vi "Configure.vi"(8 "error in (no error)":errorcluster, 10 "Msg in":T7, 11 "FakePressureController in":refnum<class "MagAnalysis_Online.lvclass">) -> (0 "error out":errorcluster, 1 "new command":string, 2 "Msg out":T7, 3 "FakePressureController out":refnum<class "MagAnalysis_Online.lvclass">)   [LabVIEW 2020, in "MagAnalysis_Online.lvclass"]
uses:
  MagAnalysis_Online.lvclass
  DriverMsg.ctl
  CamSettingSUB_TypDEf.ctl
  CamAndObj_TypDEf.ctl
  OnOffTypeDef.ctl
  userROI.ctl
  source/Device Drivers/shared/numericVariable_TypeDef.ctl
  CamRoiTypDef.ctl
  MagAnalysis_Online.lvclass/MagAnalysis_Online.ctl
  source/Device Drivers/BaseDriver/BaseDriver.lvclass
  <resource>/objmgr/imaqdx.rc
panel:
  out "found? 2":bool
  out "found?":bool
  out "Cam 2.center":dbl
  out "Cam 1.center":dbl
  out "data":T1={"position"=0.0, "pixelsize"=0.0, "start"=0.0, "end"=0.0, "center"=0.0, "Lens"=enum."FL1-f8x08", "Forward"=enum."off", "Spec_Calib_file 2"=path "Y:/100TWdata/ESMCalib/datFwd.txt", "map"=path "Y:/100TWdata/ESMCalib/mapFwd.txt", "y size"=0, "UserROI"={"Width"={"Value"=0.0, "Min"=0.0, "Max"=0.0, "StepSize"=0.0, "Tolerance"=0.0, "ValueActual"=0.0}, "Hight"={"Value"=0.0, "Min"=0.0, "Max"=0.0, "StepSize"=0.0, "Tolerance"=0.0, "ValueActual"=0.0}, "OffsetX"={"Value"=0.0, "Min"=0.0, "Max"=0.0, "StepSize"=0.0, "Tolerance"=0.0, "ValueActual"=0.0}, "OffsetY"={"Value"=0.0, "Min"=0.0, "Max"=0.0, "StepSize"=0.0, "Tolerance"=0.0, "ValueActual"=0.0}}, "CamMaxPixel"={"X"=0, "Y"=0}, "CamROI"={"Width"=0.0, "Hight"=0.0, "OffsetX"=0.0, "OffsetY"=0.0}}
  out "Cam 0.center":dbl
  out "before substring 2":string
  out "ROI":i32[][](array[numeric])
  out "number":i32
  out "Command":string
  out "Channel":string
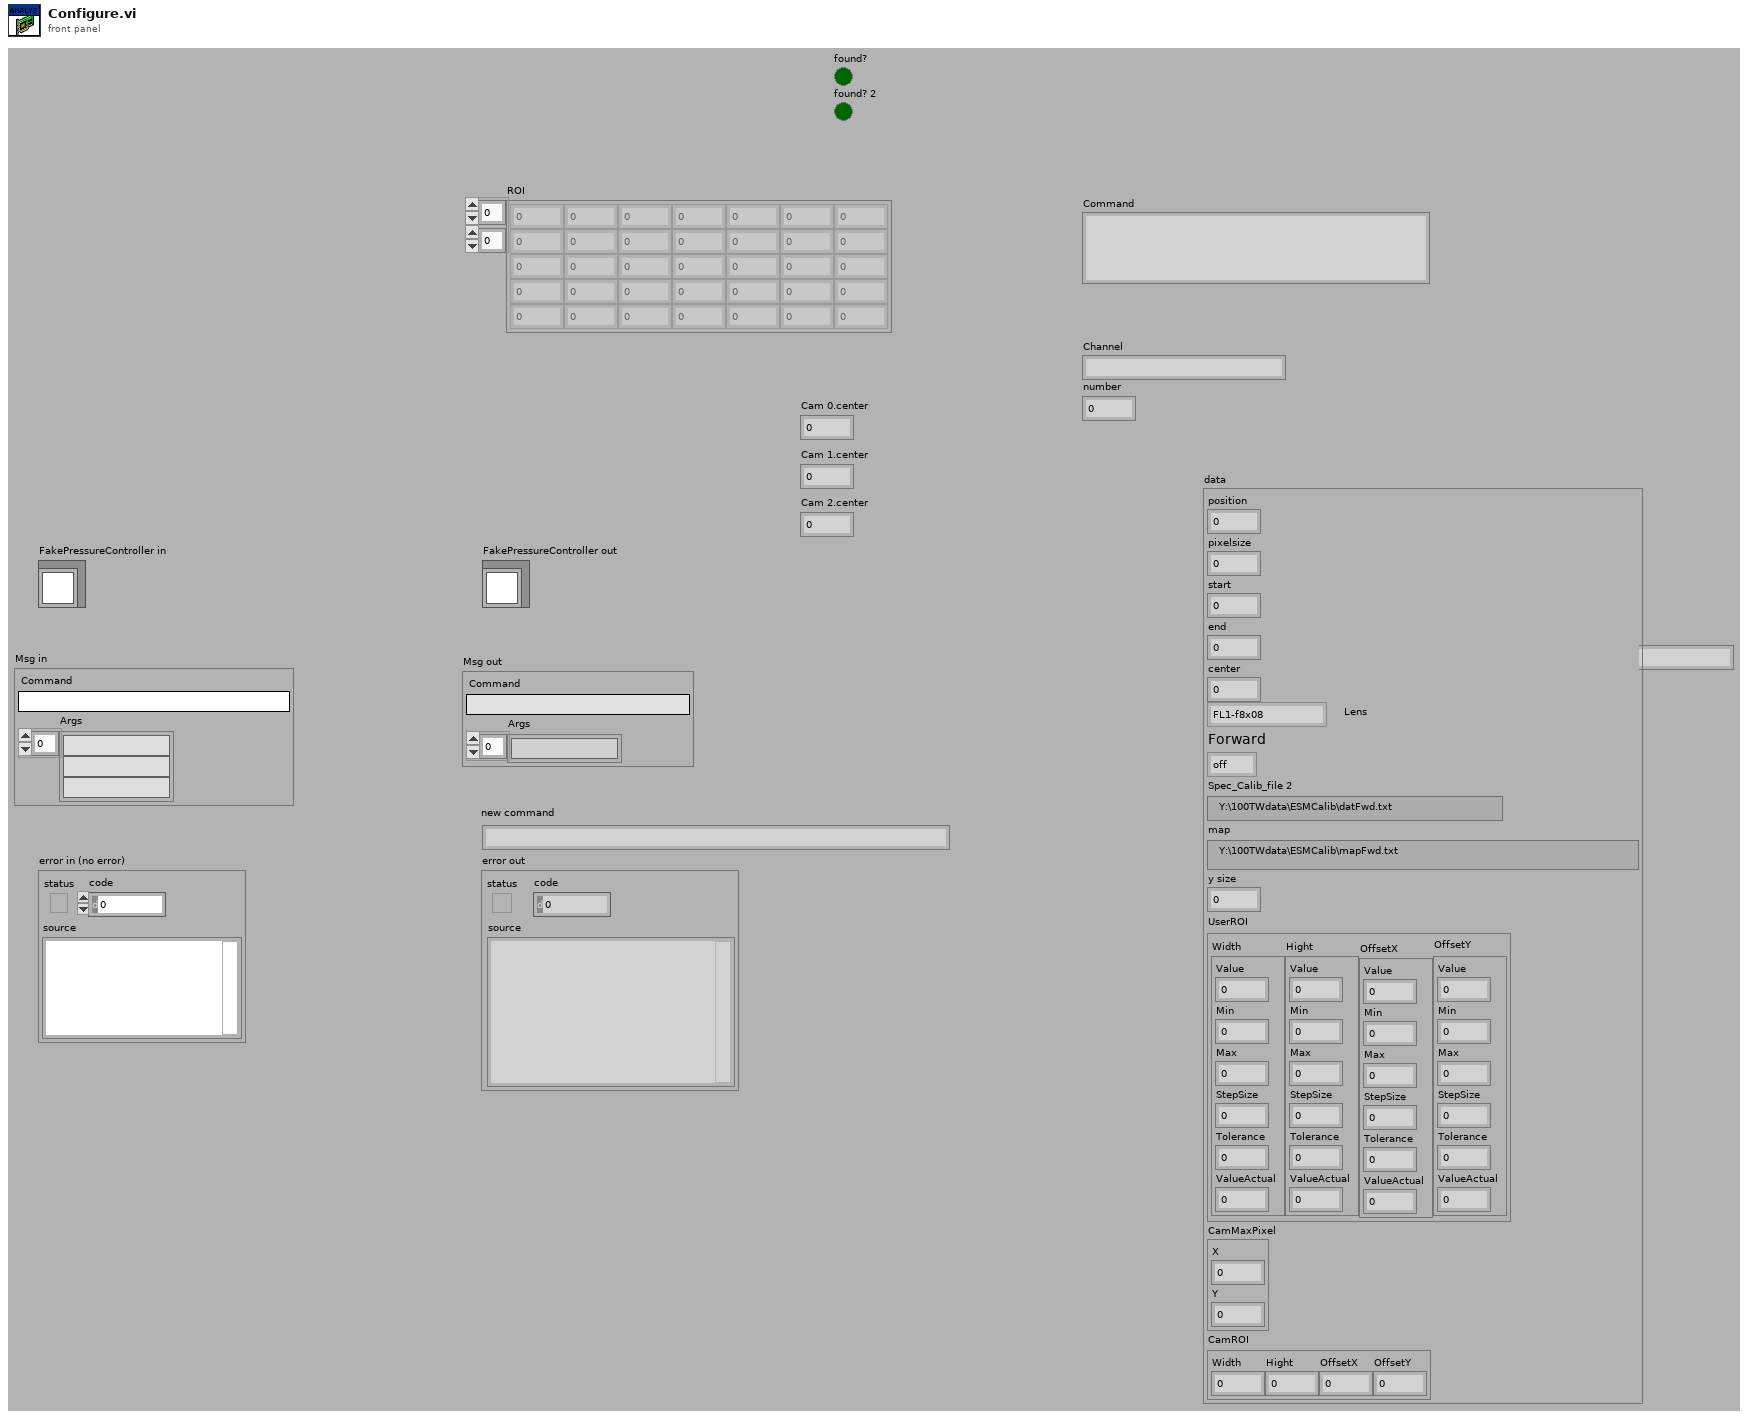
[diagram p1: front panel]
types:
  T1 = typedef "CamSettingSUB_TypDEf.ctl" = cluster{"position":dbl, "pixelsize":dbl, "start":dbl, "end":dbl, "center":dbl, "Lens":T2, "Forward":T3, "Spec_Calib_file 2":path, "map":path, "y size":i32, "UserROI":T4, "CamMaxPixel":cluster{"X":i32, "Y":i32}, "CamROI":T6}
  T2 = typedef "CamAndObj_TypDEf.ctl" = enum16{"FL1-f8x08", "FL1-f8x06", "FL1-f8", "ch300-f50", "FL2G-f8", "FL3M14-f8", "FL3M14-f8x08", "FL3M14-f8x08(2x2)"}
  T3 = typedef "OnOffTypeDef.ctl" = enum16{"off", "on"}
  T4 = typedef "userROI.ctl" = cluster{"Width":T5, "Hight":T5, "OffsetX":T5, "OffsetY":T5}
  T5 = typedef "BaseDriver.lvclass/numericVariable_TypeDef.ctl" = cluster{"Value":dbl, "Min":dbl, "Max":dbl, "StepSize":dbl, "Tolerance":dbl, "ValueActual":dbl}
  T6 = typedef "CamRoiTypDef.ctl" = cluster{"Width":dbl, "Hight":dbl, "OffsetX":dbl, "OffsetY":dbl}
  T7 = typedef "DriverMsg.ctl" = cluster{"Command":string, "Args":string[]}
  T8 = typedef "MagAnalysis_Online.lvclass/settings_TypDef.ctl" = cluster{"CamSettings":T9, "timeout":T5, "Screws":T10, "number of cam":dbl, "X size":dbl, "srewstart":T13, "Save":T3, "offset":dbl, "localsavingpath":path, "ROIString":string, "exposure":T5, "trigger":T3}
  T9 = typedef "CamSettings_Typdef.ctl" = cluster{"Cam 0":T1, "Cam 1":T1, "Cam 2":T1, "Cam 3":T1}
  T10 = typedef "SrewMaster_TYpDef.ctl" = cluster{"Cam 0":T11, "Cam 1":T11, "Cam 2":T11, "Cam 3":T11}
  T11 = typedef "srew_TypDEf.ctl" = cluster{"S 0":T12, "S 1":T12, "S 2":T12, "S 3":T12, "S 4":T12, "S 5":T12}
  T12 = typedef "ScrewSub_Typdef.ctl" = cluster{"0":i32, "1":i32, "2":i32, "3":i32}
  T13 = typedef "screwstart.ctl" = cluster{"Cam 0":dbl, "Cam 1":dbl, "Cam 2":dbl, "Cam 3":dbl}
  T14 = typedef "IMAQdx.ctl" = refnum<k21>
  T15 = cluster{"CamSettings[0]":T1, "CamSettings[1]":T1, "CamSettings[2]":T1, "CamSettings[3]":T1}
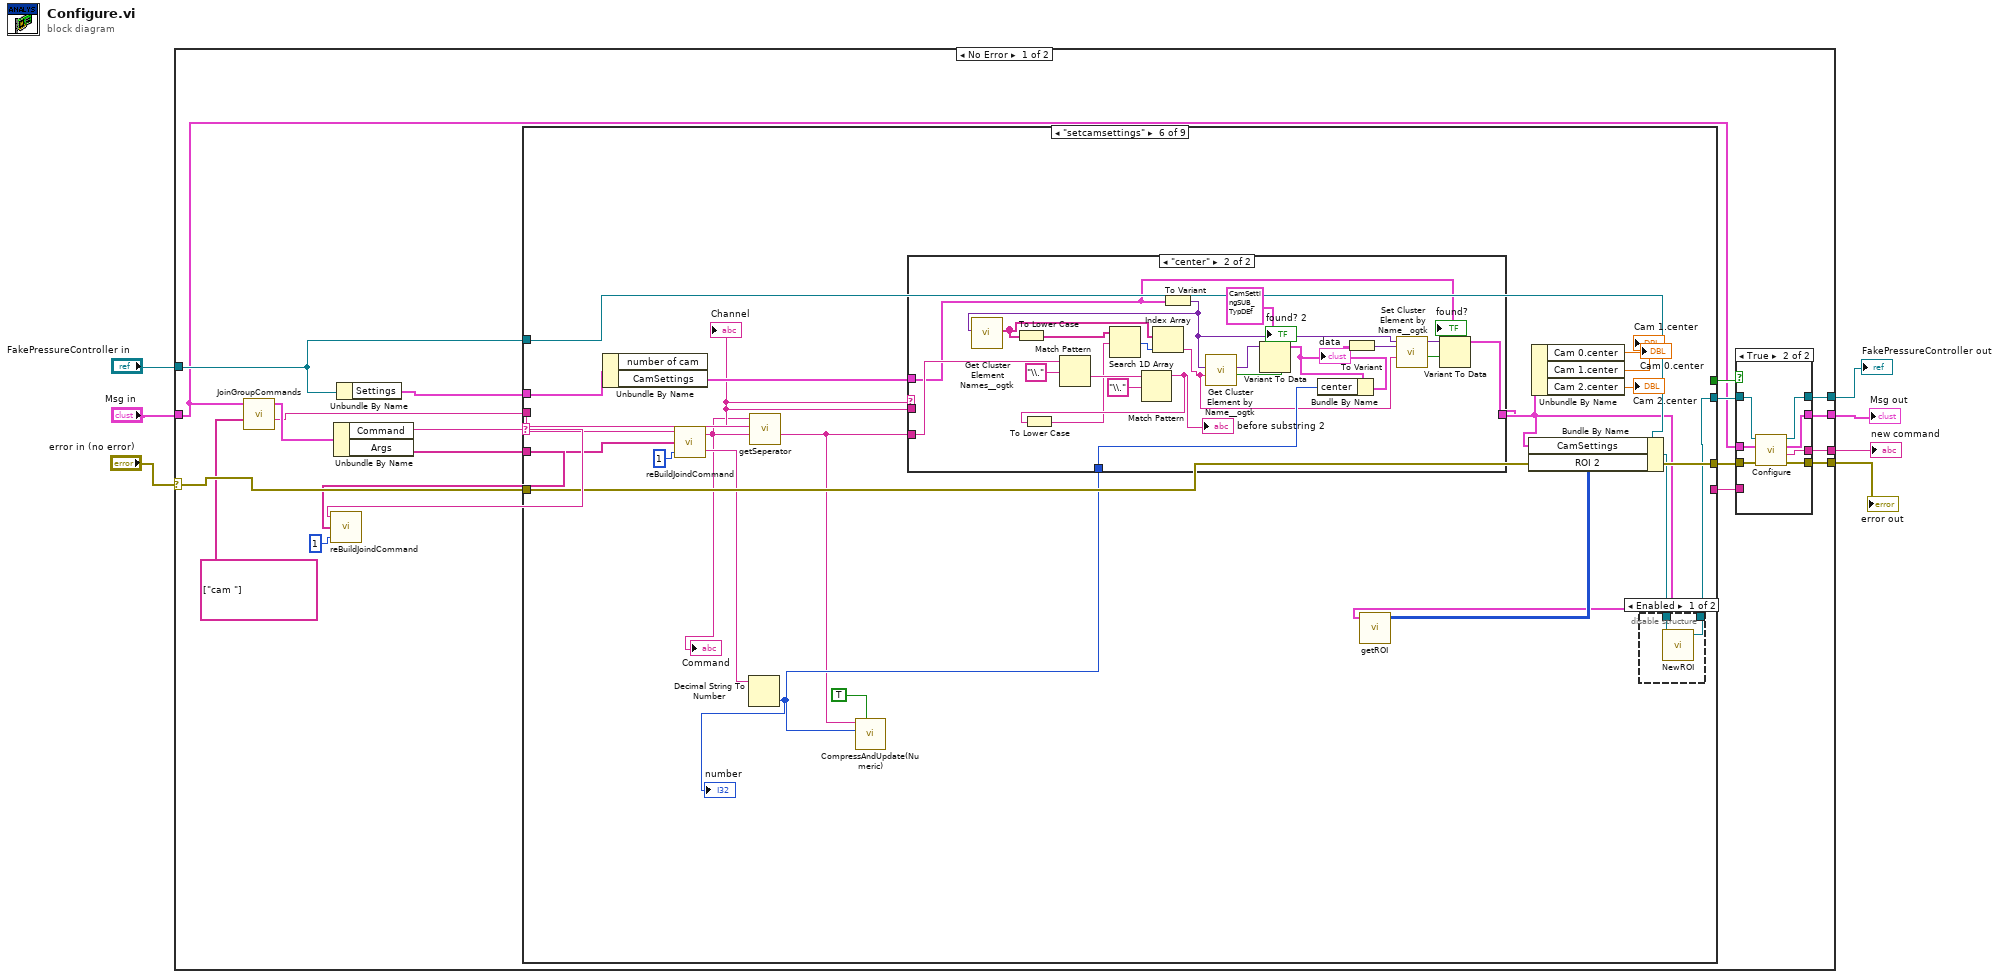
[diagram p0: block diagram]
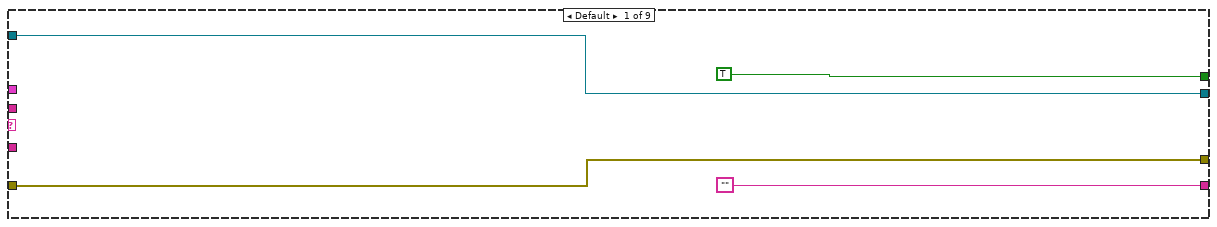
[diagram p3: hidden frame]
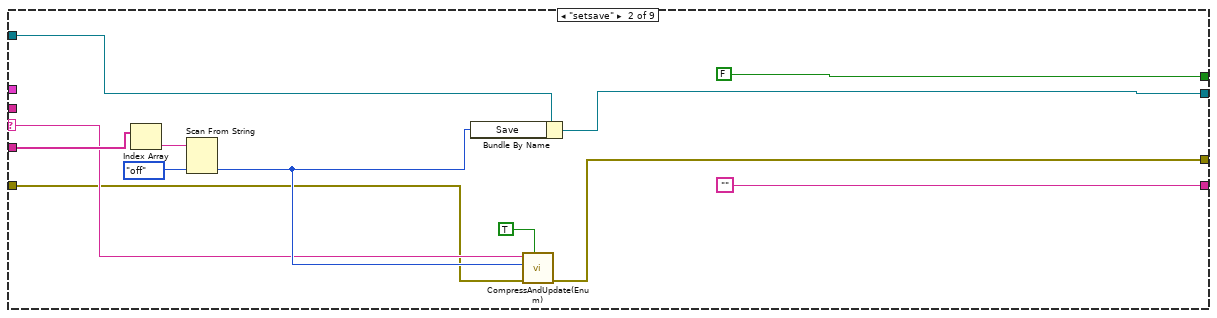
[diagram p4: hidden frame]
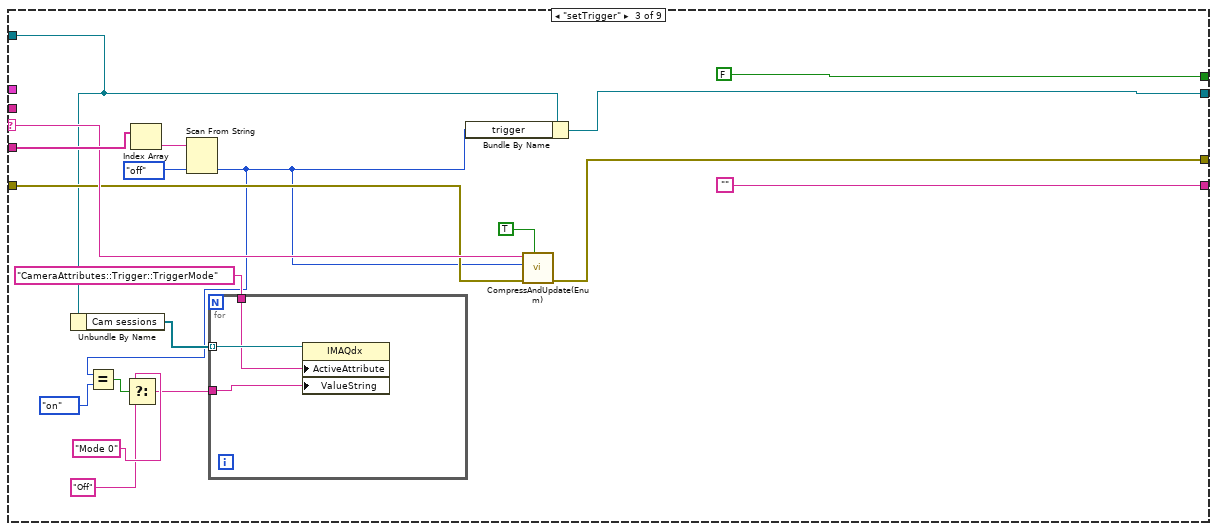
[diagram p5: hidden frame]
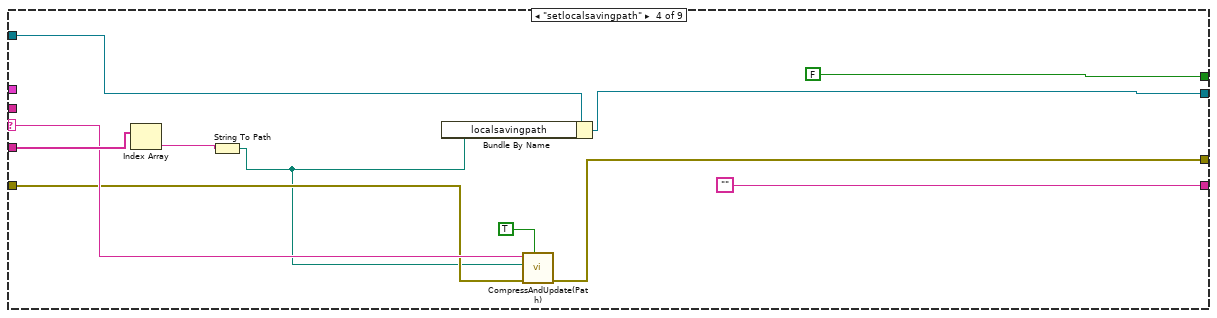
[diagram p6: hidden frame]
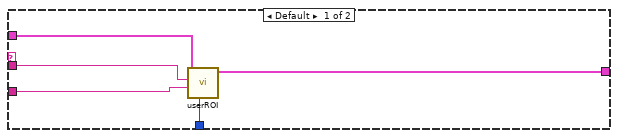
[diagram p9: hidden frame]
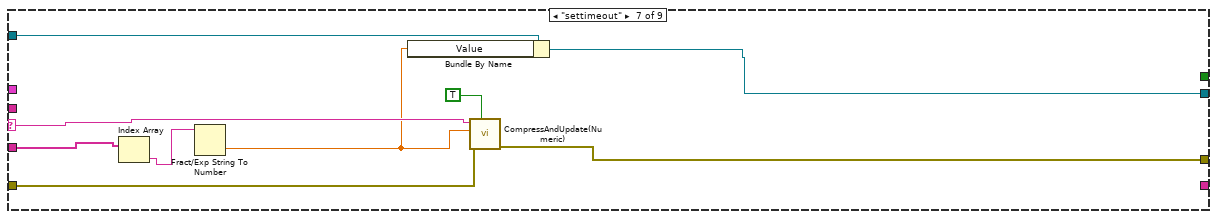
[diagram p10: hidden frame]
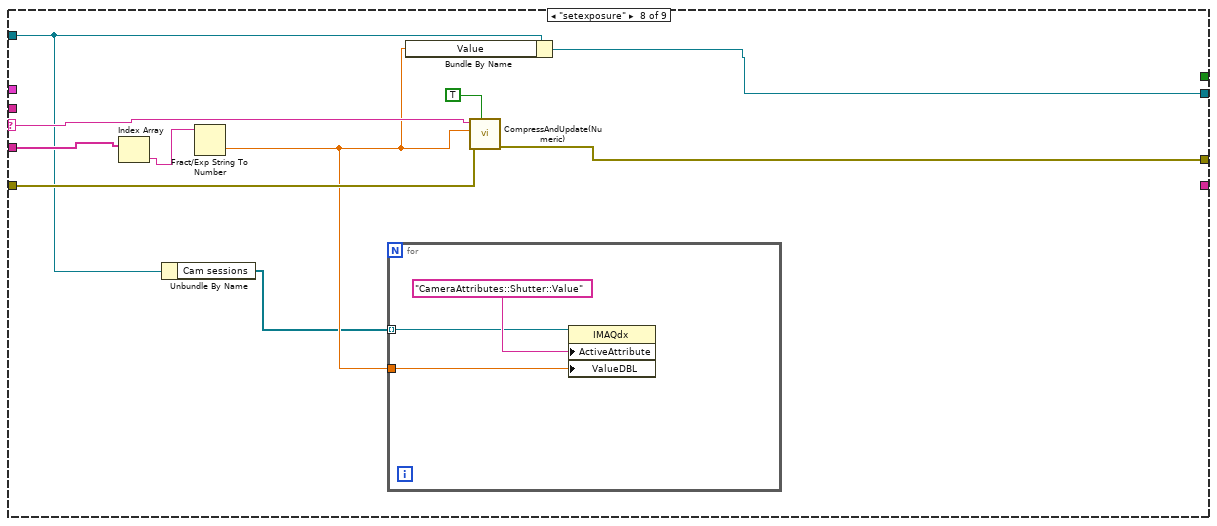
[diagram p11: hidden frame]
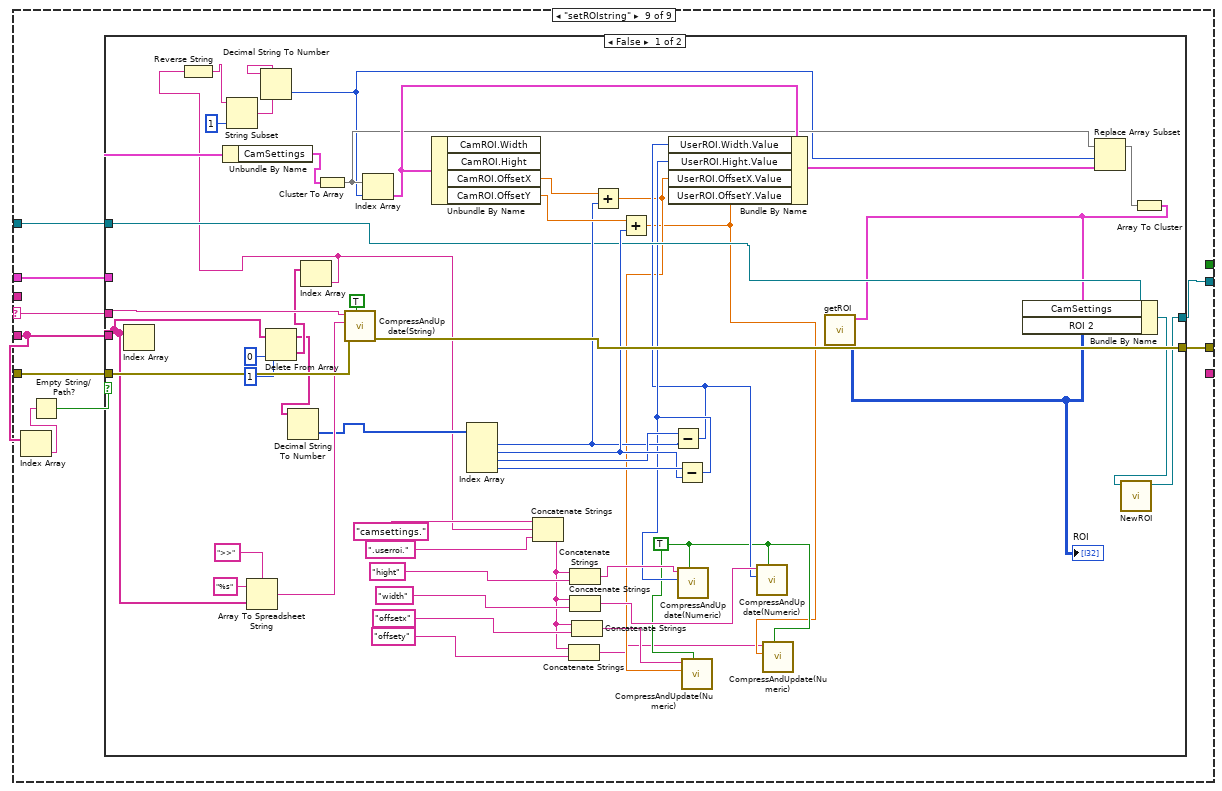
[diagram p12: hidden frame]
diagram:
  n1 = case shown="No Error" "error in (no error)" {
    selector: "error in (no error)" -> [w16 w224]
    tunnel: "FakePressureController in" -> [w17 w222]
    tunnel: [w24 w222] -> w4
    tunnel: [w22 w224] -> w1
    tunnel: "Msg in" -> [w15 w223]
    tunnel: [w20 w223] -> w3
    tunnel: [w18 _] -> w2
    frame No Error {
      n2 = call "JoinGroupCommands.vi"("Seperator between var name and chan num"=string[] ["cam "] ("Seperator"), "Msg in"=w15) -> ("Seperator out"=w9:string, "Msg out"=w14:T7)  [unwired: 6 in, 2 out]
      n3 = Unbundle By Name(w14) -> ("Command"=w11:string, "Args"=w10:string[])
      n4 = call "reBuildJoindCommand.vi"("number of group elements (0)"=1, "Args"=w10, "Command 2"=w11) -> ()  [unwired: 2 out]
      n5 = Unbundle By Name(w17) -> ("Settings"=w8:T8)
      n6 = case shown="\"setcamsettings\"" w11 {
        selector: w11 -> [_ w43 w64 w80 _ w105 w141 w152 w168]
        tunnel: w16 -> [w39 w42 w63 w79 w86 w107 w139 w151 w167]
        tunnel: w10 -> [_ w50 w69 w84 _ w104 w146 w156 w162]
        tunnel: w17 -> [w40 w47 w61 w83 w87 w99 w144 w148 w164]
        tunnel: [w40 w46 w66 w82 w87 w94 w143 w154 w163] -> w25
        tunnel: ["" ("Complete") "" ("Complete") "" ("Complete") "" ("Complete") _ _ _ _ _] -> w19
        tunnel: [w39 w41 w62 w78 w86 w107 w138 w150 w166] -> w23
        tunnel: [TRUE FALSE FALSE FALSE _ _ _ _ _] -> w21
        tunnel: w8 -> [_ _ _ _ _ w102 _ _ w165]
        tunnel: w9 -> [_ _ _ _ _ w103 _ _ _]
        frame Default {
        }
        frame "setsave" {
          n7 = Index Array(array=w50) -> (element=w49:string)  [unwired: 1 in]
          n8 = Scan From String(input string=w49, default 1=OnOffTypeDef."off" ("Save")) -> (output 1=w44:T3)  [unwired: 3 in, 3 out]
          n9 = Bundle By Name(cluster=w47, "Save"=w44) -> (w46:refnum<class "MagAnalysis_Online.lvclass">)
          n10 = call "CompressAndUpdate(Enum).vi"("force CVT update (false)"=TRUE, "error in"=w42, "enum variant"=w44, "command or variable name"=w43) -> ("error out"=w41:errorcluster)  [unwired: 7 in]
        }
        frame "setTrigger" {
          n11 = Unbundle By Name(w61) -> ("Cam sessions"=w60:T14[])
          n12 = Index Array(array=w69) -> (element=w68:string)  [unwired: 1 in]
          n13 = Scan From String(input string=w68, default 1=OnOffTypeDef."off" ("Save")) -> (output 1=w57:T3)  [unwired: 3 in, 3 out]
          n14 = Equal?(x=w57, y=OnOffTypeDef."on" ("Save")) -> (x = y?=w56:bool)
          n15 = Select(t="Mode 0", s=w56, f="Off") -> (s? t:f=w53:string)
          n16 = for {
            tunnel: w60 -> [w74] mode=indexing
            tunnel: "CameraAttributes::Trigger::TriggerMode" -> [w73]
            tunnel: w53 -> [w72]
            n17 = property class="IMAQdx"(reference=w74, "ActiveAttribute"=w73, "ValueString"=w72) -> ()  [unwired: 1 in, 2 out]
          }
          n18 = Bundle By Name(cluster=w61, "trigger"=w57) -> (w66:refnum<class "MagAnalysis_Online.lvclass">)
          n19 = call "CompressAndUpdate(Enum).vi"("force CVT update (false)"=TRUE, "error in"=w63, "enum variant"=w57, "command or variable name"=w64) -> ("error out"=w62:errorcluster)  [unwired: 7 in]
        }
        frame "setlocalsavingpath" {
          n20 = Index Array(array=w84) -> (element=w77:string)  [unwired: 1 in]
          n21 = String To Path(string=w77) -> (path=w76:path)
          n22 = Bundle By Name(cluster=w83, "localsavingpath"=w76) -> (w82:refnum<class "MagAnalysis_Online.lvclass">)
          n23 = call "CompressAndUpdate(Path).vi"("force CVT update (false)"=TRUE, "error in"=w79, "Path"=w76, "command or variable name"=w80) -> ("error out"=w78:errorcluster)  [unwired: 7 in]
        }
        frame "Abort" {
        }
        frame "setcamsettings" {
          n24 = Unbundle By Name(w102) -> ("CamSettings"=w100:T9)  [unwired: 1 out]
          n25 = call "reBuildJoindCommand.vi"("number of group elements (0)"=1, "Args"=w104, "Command 2"=w105) -> ("Arg"=w101:string, "Command"=w92:string)
          "Command" <- w92
          n26 = Decimal String To Number(string=w101) -> (number=w97:i32)  [unwired: 2 in, 1 out]
          "number" <- w97
          n27 = call "getSeperator.vi"("Channel Seperator (\"\")"=w103, "Command"=w92) -> ("Channel"=w93:string)  [unwired: 8 in, 1 out]
          "Channel" <- w93
          n28 = call "CompressAndUpdate(Numeric).vi"("force CVT update (false)"=TRUE, "Numeric"=w97, "command or variable name"=w92) -> ()  [unwired: 8 in, 1 out]
          n29 = case shown="\"center\"" w93 {
            tunnel: w100 -> [w115 w126]
            tunnel: w92 -> [w114 w133]
            tunnel: w93 -> [w113 _]
            tunnel: w97 -> [w112 w131]
            tunnel: [w111 w125] -> w91
            frame Default {
              n30 = call "userROI.vi"("Numeric"=w112, "Command"=w114, "Channel"=w113, "CamSettings in"=w115) -> ("CamSettings out"=w111:T9)  [unwired: 6 in, 1 out]
            }
            frame "center" {
              n31 = Match Pattern(string=w133, regular expression="\\.") -> (after substring=w135:string)  [unwired: 1 in, 3 out]
              n32 = Match Pattern(string=w135, regular expression="\\.") -> (before substring=w123:string)  [unwired: 1 in, 3 out]
              "before substring 2" <- w123
              n33 = To Lower Case(string=w123) -> (all lower case string=w121:string)
              n34 = To Variant(anything=w126) -> (Variant=w124:variant)
              n35 = call "Get Cluster Element Names__ogtk.vi"("Cluster"=w124) -> ("Element Names"=w120:string[])  [unwired: 9 in, 1 out]
              n36 = To Lower Case(string=w120) -> (all lower case string=w122:string[])
              n37 = Search 1D Array(1D array=w122, element=w121) -> (index of element=w119:i32)  [unwired: 1 in]
              n38 = Index Array(array=w120, index=w119) -> (element=w116:string)
              n39 = call "Get Cluster Element by Name__ogtk.vi"("Element Name"=w116, "Cluster"=w124) -> ("found?"=→"found? 2":bool, "VElement"=w128:variant)  [unwired: 7 in, 1 out]
              n40 = Variant To Data(type=T1 {"position"=0.0, "pixelsize"=0.0, "start"=0.0, "end"=0.0, "center"=0.0, "Lens"=enum."FL1-f8x08", "Forward"=enum."off", "Spec_Calib_file 2"=path "Y:/100TWdata/ESMCalib/datFwd.txt", "map"=path "Y:/100TWdata/ESMCalib/mapFwd.txt", "y size"=0, "UserROI"={"Width"={"Value"=0.0, "Min"=0.0, "Max"=0.0, "StepSize"=0.0, "Tolerance"=0.0, "ValueActual"=0.0}, "Hight"={"Value"=0.0, "Min"=0.0, "Max"=0.0, "StepSize"=0.0, "Tolerance"=0.0, "ValueActual"=0.0}, "OffsetX"={"Value"=0.0, "Min"=0.0, "Max"=0.0, "StepSize"=0.0, "Tolerance"=0.0, "ValueActual"=0.0}, "OffsetY"={"Value"=0.0, "Min"=0.0, "Max"=0.0, "StepSize"=0.0, "Tolerance"=0.0, "ValueActual"=0.0}}, "CamMaxPixel"={"X"=0, "Y"=0}, "CamROI"={"Width"=0.0, "Hight"=0.0, "OffsetX"=0.0, "OffsetY"=0.0}} ("Cam 0"), Variant=w128) -> (data=w132:T1)  [unwired: 1 in, 1 out]
              "data" <- w132
              n41 = Bundle By Name(cluster=w132, "center"=w131) -> (w130:T1)
              n42 = To Variant(anything=w130) -> (Variant=w129:variant)
              n43 = call "Set Cluster Element by Name__ogtk.vi"("Element Name (\"\": New Element Data Name)"=w116, "New Element Value"=w129, "Cluster"=w124) -> ("found?"=→"found?":bool, "VCluster out"=w127:variant)  [unwired: 6 in, 1 out]
              n44 = Variant To Data(type=w126, Variant=w127) -> (data=w125:T9)  [unwired: 1 in, 1 out]
            }
          }
          n45 = call "getROI.vi"("CamSettings"=w91) -> ("ROI"=w96:i32[][])  [unwired: 10 in]
          n46 = Bundle By Name(cluster=w99, "CamSettings"=w91, "ROI 2"=w96) -> (w95:refnum<class "MagAnalysis_Online.lvclass">)
          n47 = Unbundle By Name(w91) -> ("Cam 0.center"=→"Cam 0.center":dbl, "Cam 1.center"=→"Cam 1.center":dbl, "Cam 2.center"=→"Cam 2.center":dbl)
          n48 = disable-structure shown="Enabled" {
            disable-tunnel: w95 -> [w109 w110]
            disable-tunnel: [w108 w110] -> w94
            frame Enabled {
              n49 = call "NewROI.vi"("MagAnalysis_Online in"=w109) -> ("MagAnalysis_Online out"=w108:refnum<class "MagAnalysis_Online.lvclass">)  [unwired: 10 in]
            }
            frame Disabled {
            }
          }
        }
        frame "settimeout" {
          n50 = Index Array(array=w146) -> (element=w145:string)  [unwired: 1 in]
          n51 = Fract/Exp String To Number(string=w145) -> (number=w140:dbl)  [unwired: 3 in, 1 out]
          n52 = Bundle By Name(cluster=w144, "Value"=w140) -> (w143:refnum<class "MagAnalysis_Online.lvclass">)
          n53 = call "CompressAndUpdate(Numeric).vi"("force CVT update (false)"=TRUE, "error in"=w139, "Numeric"=w140, "command or variable name"=w141) -> ("error out"=w138:errorcluster)  [unwired: 7 in]
        }
        frame "setexposure" {
          n54 = Index Array(array=w156) -> (element=w155:string)  [unwired: 1 in]
          n55 = Unbundle By Name(w148) -> ("Cam sessions"=w147:T14[])
          n56 = Fract/Exp String To Number(string=w155) -> (number=w149:dbl)  [unwired: 3 in, 1 out]
          n57 = for {
            tunnel: w149 -> [w158]
            tunnel: w147 -> [w157] mode=indexing
            n58 = property class="IMAQdx"(reference=w157, "ActiveAttribute"="CameraAttributes::Shutter::Value", "ValueDBL"=w158) -> ()  [unwired: 1 in, 2 out]
          }
          n59 = Bundle By Name(cluster=w148, "Value"=w149) -> (w154:refnum<class "MagAnalysis_Online.lvclass">)
          n60 = call "CompressAndUpdate(Numeric).vi"("force CVT update (false)"=TRUE, "error in"=w151, "Numeric"=w149, "command or variable name"=w152) -> ("error out"=w150:errorcluster)  [unwired: 7 in]
        }
        frame "setROIstring" {
          n61 = Index Array(array=w162) -> (element=w161:string)  [unwired: 1 in]
          n62 = Empty String/Path?(string/path=w161) -> (empty?=w160:bool)
          n63 = case shown="False" w160 {
            tunnel: w168 -> [w218 _]
            tunnel: w167 -> [w217 w221]
            tunnel: [w216 w221] -> w166
            tunnel: w165 -> [w212 _]
            tunnel: w162 -> [w206 _]
            tunnel: w164 -> [w190 w220]
            tunnel: [w170 w220] -> w163
            frame False {
              w177 = TRUE ("force CVT update (false)")
              n64 = Index Array(array=w206) -> ()  [unwired: 1 in, 1 out]
              n65 = Unbundle By Name(w212) -> ("CamSettings"=w208:T9)
              n66 = Array To Spreadsheet String(delimiter (Tab)=">>", array=w206, 3:"%s" ("format string")) -> (spreadsheet string=w213:string)
              n67 = Delete From Array(array=w206, length=1, index=0) -> (deleted portion=w203:string[], array with subset deleted=w202:string[])
              n68 = Decimal String To Number(string=w202) -> (number=w201:i32[])  [unwired: 2 in, 1 out]
              n69 = Index Array(array=w203) -> (element=w188:string)  [unwired: 1 in]
              n70 = Reverse String(1:w188) -> (0:w209:string)
              n71 = String Subset(string=w209, length (rest)=1 ("length (rest)")) -> (substring=w211:string)  [unwired: 1 in]
              n72 = Decimal String To Number(string=w211) -> (number=w193:i32)  [unwired: 2 in, 1 out]
              n73 = Cluster To Array(cluster=w208) -> (array=w194:T1[])
              n74 = call "CompressAndUpdate(String).vi"("force CVT update (false)"=TRUE, "error in"=w217, "String"=w213, "command or variable name"=w218) -> ("error out"=w216:errorcluster)  [unwired: 7 in]
              n75 = Index Array(array=w194, index=w193) -> (element=w207:T1)
              n76 = Unbundle By Name(w207) -> ("CamROI.OffsetX"=w200:dbl, "CamROI.OffsetY"=w199:dbl)  [unwired: 2 out]
              n77 = Index Array(array=w201) -> (element #1=w195:i32, element #2=w197:i32, element #3=w196:i32, element #4=w198:i32)  [unwired: 4 in]
              n78 = Concatenate Strings("camsettings.", w188, ".userroi.") -> (w183:string)
              n79 = Concatenate Strings(w183, "offsety") -> (w173:string)
              n80 = Concatenate Strings(w183, "hight") -> (w181:string)
              n81 = Concatenate Strings(w183, "width") -> (w180:string)
              n82 = Concatenate Strings(w183, "offsetx") -> (w176:string)
              n83 = Add(x=w200, y=w195) -> (x+y=w175:dbl)
              n84 = Add(x=w199, y=w197) -> (x+y=w174:dbl)
              n85 = Subtract(x=w196, y=w195) -> (x-y=w178:i32)
              n86 = Subtract(x=w198, y=w197) -> (x-y=w179:i32)
              n87 = Bundle By Name(cluster=w207, "UserROI.Width.Value"=w178, "UserROI.Hight.Value"=w179, "UserROI.OffsetX.Value"=w175, "UserROI.OffsetY.Value"=w174) -> (w192:T1)
              n88 = call "CompressAndUpdate(Numeric).vi"("force CVT update (false)"=w177, "Numeric"=w179, "command or variable name"=w181) -> ()  [unwired: 8 in, 1 out]
              n89 = call "CompressAndUpdate(Numeric).vi"("force CVT update (false)"=w177, "Numeric"=w175, "command or variable name"=w176) -> ()  [unwired: 8 in, 1 out]
              n90 = call "CompressAndUpdate(Numeric).vi"("force CVT update (false)"=w177, "Numeric"=w178, "command or variable name"=w180) -> ()  [unwired: 8 in, 1 out]
              n91 = call "CompressAndUpdate(Numeric).vi"("force CVT update (false)"=w177, "Numeric"=w174, "command or variable name"=w173) -> ()  [unwired: 8 in, 1 out]
              n92 = Replace Array Subset(array=w194, new element=w192, index=w193) -> (w191:T1[])
              n93 = Array To Cluster(array=w191) -> (cluster=w172:T15)
              n94 = call "getROI.vi"("CamSettings"=w172) -> ("ROI"=w169:i32[][])  [unwired: 10 in]
              "ROI" <- w169
              n95 = Bundle By Name(cluster=w190, "CamSettings"=w172, "ROI 2"=w169) -> (w171:refnum<class "MagAnalysis_Online.lvclass">)
              n96 = call "NewROI.vi"("MagAnalysis_Online in"=w171) -> ("MagAnalysis_Online out"=w170:refnum<class "MagAnalysis_Online.lvclass">)  [unwired: 10 in]
            }
            frame True {
            }
          }
        }
      }
      n97 = case shown="True" w21 {
        tunnel: w25 -> [w27 w36]
        tunnel: [w27 w35] -> w24
        tunnel: [w28 w34] -> w18
        tunnel: w23 -> [w26 w33]
        tunnel: [w26 w32] -> w22
        tunnel: w15 -> [w29 w31]
        tunnel: [w29 w30] -> w20
        tunnel: w19 -> [w28 _]
        frame False {
        }
        frame True {
          n98 = call-parent "Configure.vi"("error in (no error)"=w33, "Msg in"=w31, "BaseDriver in"=w36) -> ("error out"=w32:errorcluster, "new command"=w34:string, "Msg out"=w30:T7, "BaseDriver out"=w35:refnum<class "MagAnalysis_Online.lvclass">)  [unwired: 5 in]
        }
      }
    }
    frame Error {
    }
  }
  "error out" <- w1
  "FakePressureController out" <- w4
  "new command" <- w2
  "Msg out" <- w3
